vi "DivergeAngleScan.vi"(6 "Backgrund":T1, 7 "Session In":T2, 8 "俯仰CCD0":dbl, 10 "激光出口至CCD距离":dbl, 11 "旋转CCD0":dbl) -> (2 "近场图像":T1(plugin-control))   [LabVIEW 2018]
uses:
  <vilib>/userdefined/High Color/IMAQdx.ctl
  <vilib>/vision/Image Controls.llb/IMAQ Image.ctl
  <vilib>/vision/NI_Vision_Development_Module.lvlib
  <vilib>/vision/driver/NI_Vision_Acquisition_Software.lvlib
panel:
  out "近场相机.近场X范围":dbl
  out "近场相机.近场Y范围":dbl
  in  "停止":bool
  out "进度":dbl format="%05.2f%"
  out "YResolution":i32
  out "X Resolution":i32
  out "采集时间":u32
  out "运动时间":u32
  out "总时间":u32
  out "单步时间":u32
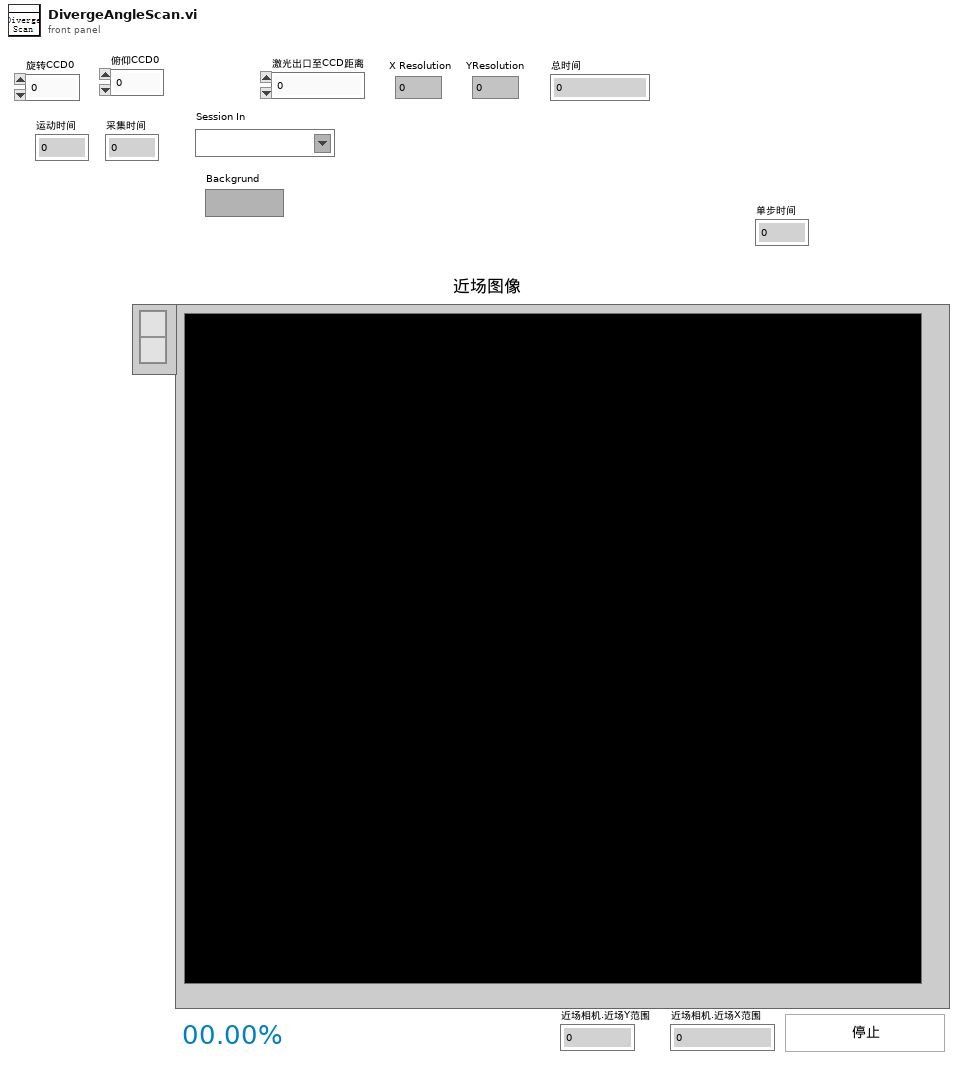
[diagram p1: front panel]
types:
  T1 = typedef "IMAQ Image.ctl" = refnum<image>
  T2 = typedef "IMAQdx.ctl" = refnum<k21>
  T3 = enum16{"计算总分辨率", "计算偏移量", "计算发散角分辨率", "计算发散角偏移量"}
  T4 = typedef "Image Type" = u32
  T5 = cluster{"示波器":cluster{"Channel (0:Channel 1)":enum16{"Channel 1", "Channel 2", "Channel 3", "Channel 4"}, "电压范围":dbl, "触发电压":dbl, "时间范围":dbl, " 示波器VISA":refnum<visa-resource-name>, "时间范围 标签":u64, "电压范围 标签":u64, "触发电压 标签":u64, "输入阻抗/Ω":u64}, "光谱仪":cluster{"SpecDataReference":refnum<queue>, "grating center":dbl, "Exposure Time (s)":dbl, "是否进行详细设置":bool, " 开始通信检查":bool, "通信成功？":bool, "波长":dbl}, " 近场相机":cluster{"曝光时间/us":dbl, "模拟增益":i32, "控制套接字":i32, "IP 地址":string, " 采集套接字":i32, "  版本号":i32, "ImageData":T1, "  增益最大":i32, "  增益最小":i32, " 曝光最大":i32, " 曝光最小":i32, " 帧速":i32, " 同步切换":i32, "  曝光缩放":i32, "Camera Source":refnum<k21>, "近场X范围":dbl, "近场Y范围":dbl, "单个像元大小/um":dbl, "相机距离原点位置":dbl[], "是否测量发散角":bool, "光束类型":bool}, " 偏振仪":cluster{"电压范围":u64, "触发电压":u64, "时间范围":u64, "波长范围":enum16{"可见光 400-700nm", "近红外 700-1100nm"}, "可见光偏振测量仪VISA":refnum<visa-resource-name>, "近红外偏振测量仪VISA":refnum<visa-resource-name>}, " 功率计":cluster{"通道":enum16{"Channel 1", "Channel 2"}, "工作波长":u32, "单位":u64, "时间范围":u64, "IP地址":string, "端口":u32, "是否需要散射片":bool}, "能量计":cluster{"通道":enum16{"Channel 1", "Channel 2"}, "工作波长":u32, "单位":u64, "时间范围":u64, "IP地址":string, "端口":u32, "能量计量程":enum16{"200uJ", "20uJ", "2uJ", "200nJ"}}, "电机":cluster{"Channel (0:Channel 1)":enum16{"Channel 1", "Channel 2", "Channel 3", "Channel 4"}, "电压范围":u64, "触发电压":u64, "时间范围":u64}, " 远场相机":cluster{"曝光时间":i32, "模拟增益":i32, "控制套接字":i32, "IP 地址":string, " 采集套接字":i32, "  版本号":i32, "ImageData":T1, "  增益最大":i32, "  增益最小":i32, " 曝光最大":i32, " 曝光最小":i32, " 帧速":i32, " 同步切换":i32, "  曝光缩放":i32, "ImageData B":T1}}
  T6 = typedef "控制电机枚举器.ctl" = enum16{"Z", "Y", "X", "发散角", "俯仰", "旋转"}
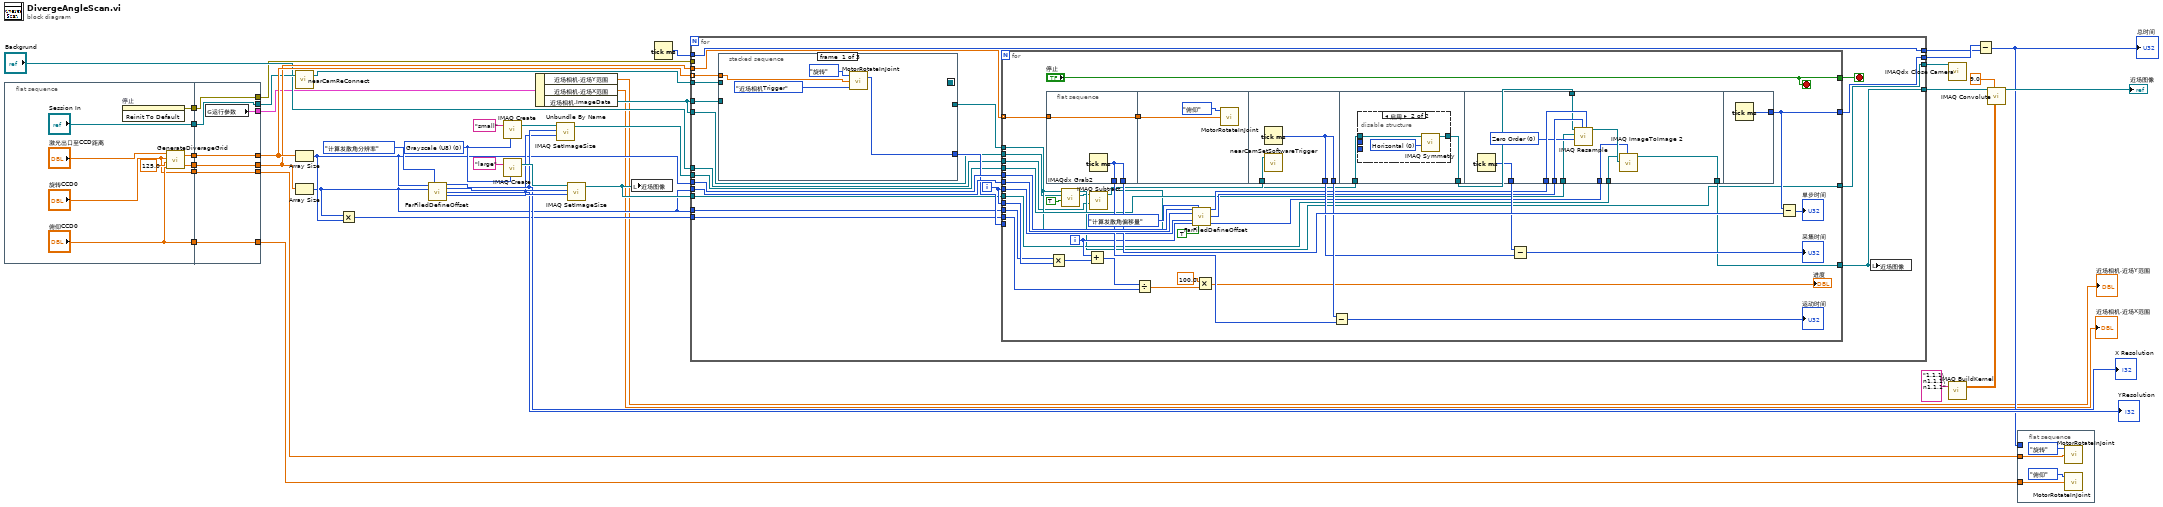
[diagram p0: block diagram]
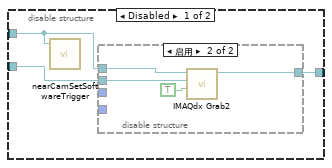
[diagram p4: hidden frame]
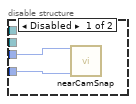
[diagram p5: hidden frame]
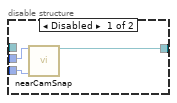
[diagram p6: hidden frame]
diagram:
  w28 = T4 0 items=["Grayscale (U8)", "Grayscale (I16)", "Grayscale (SGL)", "Complex (CSG)", "RGB (U32)", "HSL (U32)", "RGB (U64)", "Grayscale (U16)"] ("Image Type")
  n1 = flat-sequence {
    tunnel: [w49] -> w7
    tunnel: [w48] -> w6
    tunnel: ["俯仰CCD0"] -> w5
    tunnel: ["旋转CCD0"] -> w4
    tunnel: ["Session In"] -> w3
    tunnel: [w44] -> w2
    tunnel: [w53] -> w8
    tunnel: [w54] -> w13
    tunnel: [w55] -> w17
    tunnel: [w56] -> w18
    tunnel: [w57] -> w42
    tunnel: [w58] -> w43
    tunnel: w7 -> [w58]
    tunnel: w6 -> [w57]
    tunnel: w5 -> [w56]
    tunnel: w4 -> [w55]
    tunnel: w3 -> [w54]
    tunnel: w2 -> [w53]
    tunnel: [w52] -> w1
    frame #0 {
      n2 = invoke on="停止" class="Bool" method="Reinit To Default"() -> (error out=w44:errorcluster)  [unwired: 3 in, 2 out]
      n3 = call "GenerateDiverageGrid.vi"("俯仰CCD0"="俯仰CCD0", "TargetTheta"=125.0, "旋转CCD0"="旋转CCD0", "L"="激光出口至CCD距离") -> ("PitchGrid"=w48:dbl[], "RollGrid"=w49:dbl[])
    }
    frame #1 {
      n4 = global read "参数.vi" "运行参数"() -> (w52:T5)
    }
  }
  n5 = call "nearCamReConnect.vi"("Session In"=w13) -> ("IMAQdx Session Out"=w12:T2)  [unwired: 1 in, 1 out]
  n6 = Array Size(array=w43) -> (size(s)=w16:i32)
  n7 = Array Size(array=w42) -> (size(s)=w14:i32)
  n8 = Multiply(x=w14, y=w16) -> (x*y=w15:i32)
  n9 = call "FarFiledDefineOffset.vi"("X Pos Num"=w16, "状态"=T3."计算发散角分辨率", "Y Pos Num"=w14) -> ("单个分辨率X"=w21:i32, "X Resolution"=w39:i32, "单个分辨率Y"=w20:i32, "Y Resolution"=w38:i32)  [unwired: 8 in, 1 out]
  "X Resolution" <- w21
  "YResolution" <- w20
  n10 = call "IMAQ Create"("Image Name"="small", "Image Type"=w28) -> ("New Image"=w36:T1)  [unwired: 3 in, 1 out]
  n11 = call "IMAQ Create"("Image Name"="large", "Image Type"=w28) -> ("New Image"=w41:T1)  [unwired: 3 in, 1 out]
  n12 = Unbundle By Name(w1) -> ("近场相机.近场Y范围"=→"近场相机.近场Y范围":dbl, "近场相机.近场X范围"=→"近场相机.近场X范围":dbl, "近场相机.ImageData"=w22:T1)
  n13 = call "IMAQ SetImageSize"("Y Resolution"=w20, "X Resolution"=w21, "Image"=w36) -> ("Image Out"=w27:T1)  [unwired: 2 in, 1 out]
  n14 = call "IMAQ SetImageSize"("Y Resolution"=w38, "X Resolution"=w39, "Image"=w41) -> ("Image Out"=w24:T1)  [unwired: 2 in, 1 out]
  n15 = local write "近场图像"(w24) -> ()
  n16 = Tick Count (ms)() -> (millisecond timer value=w35:u32)
  n17 = for {
    tunnel: w43 -> [w68] mode=indexing
    tunnel: w42 -> [w67]
    tunnel: w27 -> [w61]
    tunnel: w24 -> [w60]
    tunnel: w16 -> [w78]
    tunnel: w14 -> [w77]
    tunnel: w35 -> [w75]
    tunnel: [w76] -> w34
    tunnel: [w75] -> w33
    tunnel: [w74] -> w29
    tunnel: w22 -> [w72]
    tunnel: [w71] -> w23
    tunnel: w12 -> [w70]
    tunnel: w22 -> [w69]
    tunnel: w15 -> [w65]
    tunnel: w14 -> [w63]
    tunnel: w8 -> [_]
    tunnel: "Backgrund" -> [w59]
    i -> [w64]
    stop <- w66 stop-if-true
    n18 = stacked-sequence {
      seq-local: [_ w83 _] -> [_ _ w84]
      tunnel: w68 -> [w81 _ _]
      tunnel: [w79 _ _] -> w73
      tunnel: w70 -> [_ w83 _]
      tunnel: w69 -> [_ _ w86]
      tunnel: [_ _ w85] -> w62
      frame #0 {
        n19 = call "MotorRotateInJoint.vi"("动作IO"=enum16{"近场相机Trigger", "远场相机Trigger"}."近场相机Trigger", "位置"=w81, "axis"=控制电机枚举器."旋转" ("控制电机")) -> ("返回"=w79:i32)  [unwired: 1 in]
      }
      frame #1 {
      }
      frame #2 {
        n20 = disable-structure shown="启用" {
          disable-tunnel: w86 -> [w89 _]
          disable-tunnel: [w88 w97] -> w85
          disable-tunnel: w84 -> [w87 w97]
          frame Disabled {
            n21 = call "nearCamSetSoftwareTrigger.vi"("IMAQdx Session"=w87) -> ()  [unwired: 3 in, 2 out]
            n22 = disable-structure shown="启用" {
              disable-tunnel: _ -> [w92 _]
              disable-tunnel: _ -> [w91 _]
              disable-tunnel: w89 -> [_ w96]
              disable-tunnel: w87 -> [_ w94]
              disable-tunnel: [_ w93] -> w88
              frame Disabled {
                n23 = call "nearCamSnap.vi"("采集套接字"=w92, "版本号"=w91) -> ("ImageData"=w90:T1)  [unwired: 9 in, 4 out]
              }
              frame Enabled {
                n24 = call <vilib>:"IMAQdx Grab2.vi"("Wait for Next Buffer? (Yes)"=TRUE, "Image In"=w96, "Session In"=w94) -> ("Session Out"=w93:T2)  [unwired: 5 in, 3 out]
              }
            }
          }
          frame Enabled {
          }
        }
      }
    }
    n25 = for {
      tunnel: w78 -> [w137]
      tunnel: w77 -> [w136]
      tunnel: w64 -> [w122]
      tunnel: [w105] -> w74
      tunnel: [w133] -> w76
      tunnel: w73 -> [_]
      tunnel: w72 -> [w101]
      tunnel: [w102] -> w71
      tunnel: w67 -> [w123] mode=indexing
      tunnel: ["停止"] -> w66
      tunnel: w65 -> [w120]
      tunnel: w64 -> [w119]
      tunnel: w63 -> [w118]
      tunnel: w62 -> [w103]
      tunnel: w61 -> [w109]
      tunnel: w60 -> [w106]
      tunnel: w59 -> [w98]
      i -> [w116]
      stop <- "停止" stop-if-true
      n26 = flat-sequence {
        tunnel: w123 -> [w139]
        tunnel: [w139] -> w135
        tunnel: [w138] -> w134
        tunnel: [w138] -> w128
        tunnel: w135 -> [w140]
        tunnel: [w143] -> w129
        tunnel: [w143] -> w125
        tunnel: w103 -> [w142]
        tunnel: [w145] -> w108
        tunnel: w99 -> [w144]
        tunnel: [w161] -> w126
        tunnel: w111 -> [w159]
        tunnel: w110 -> [w158]
        tunnel: w109 -> [w156]
        tunnel: w108 -> [w155]
        tunnel: w107 -> [w154]
        tunnel: w106 -> [w153]
        tunnel: [w152] -> w105
        tunnel: [w162] -> w133
        frame #0 {
          n27 = Tick Count (ms)() -> (millisecond timer value=w138:u32)
        }
        frame #1 {
          n28 = call "MotorRotateInJoint.vi"("位置"=w140, "axis"=控制电机枚举器."俯仰" ("控制电机")) -> ()  [unwired: 2 in, 1 out]
        }
        frame #2 {
          n29 = Tick Count (ms)() -> (millisecond timer value=w143:u32)
          n30 = call "nearCamSetSoftwareTrigger.vi"("IMAQdx Session"=w142) -> ()  [unwired: 3 in, 2 out]
        }
        frame #3 {
          n31 = disable-structure shown="启用" {
            disable-tunnel: [w148 w150] -> w145
            disable-tunnel: _ -> [w147 _]
            disable-tunnel: _ -> [w146 _]
            disable-tunnel: w144 -> [_ w149]
            frame Disabled {
              n32 = call "nearCamSnap.vi"("采集套接字"=w147, "版本号"=w146) -> ("Image Out"=w148:T1)  [unwired: 10 in, 3 out]
            }
            frame Enabled {
              w151 = u32 0 items=["Horizontal", "Vertical", "Central", "1st Diagonal", "2nd Diagonal"] ("Type of Symmetry")
              n33 = call "IMAQ Symmetry"("Type of Symmetry"=w151, "Image Src"=w149) -> ("Image Dst Out"=w150:T1)  [unwired: 3 in, 1 out]
            }
          }
        }
        frame #4 {
          w157 = u32 0 items=["Zero Order", "Bi-Linear", "Quadratic", "Cubic Spline"] ("Interpolation Type")
          n34 = Tick Count (ms)() -> (millisecond timer value=w161:u32)
          n35 = call "IMAQ Resample"("X Resolution"=w159, "Y Resolution"=w158, "Interpolation Type"=w157, "Image Dst"=w156, "Image Src"=w155) -> ("Image Dst Out"=w160:T1)  [unwired: 5 in, 1 out]
          n36 = call "IMAQ ImageToImage 2"("Offset Left/Top"=w154, "Image Src (Small)"=w160, "Image Src (Large)"=w153) -> ("Image Dst Out"=w152:T1)  [unwired: 7 in, 1 out]
        }
        frame #5 {
          n37 = Tick Count (ms)() -> (millisecond timer value=w162:u32)
        }
      }
      n38 = Multiply(x=w118, y=w119) -> (x*y=w117:i32)
      n39 = call <vilib>:"IMAQdx Grab2.vi"("Wait for Next Buffer? (Yes)"=TRUE, "Image In"=w101, "Session In"=w103) -> ("Image Out"=w100:T1, "Session Out"=w102:T2)  [unwired: 5 in, 2 out]
      n40 = Add(x=w116, y=w117) -> (x+y=w115:i32)
      n41 = call "IMAQ Subtract"("Image Src A"=w100, "Image Src B"=w98) -> ("Image Dst Out"=w99:T1)  [unwired: 5 in, 1 out]
      n42 = Divide(x=w115, y=w120) -> (x/y=w114:dbl)
      n43 = call "FarFiledDefineOffset.vi"("X Pos Num"=w137, "状态"=T3."计算发散角偏移量", "Y Pos Num"=w136, "当前X位置"=w122, "当前Y位置"=w116, "正序？"=TRUE) -> ("单个分辨率X"=w111:i32, "单个分辨率Y"=w110:i32, "offset"=w107:i32[])  [unwired: 5 in, 2 out]
      n44 = Multiply(x=100.0, y=w114) -> (x*y=→"进度":dbl)
      n45 = Subtract(x=w129, y=w128) -> (x-y=→"运动时间":u32)
      n46 = Subtract(x=w126, y=w125) -> (x-y=→"采集时间":u32)
      n47 = Subtract(x=w133, y=w134) -> (x-y=→"单步时间":u32)
    }
    n48 = local write "近场图像"(w74) -> ()
  }
  n49 = call <vilib>:"IMAQdx Close Camera.vi"("Session In"=w23) -> ()  [unwired: 10 in, 1 out]
  n50 = call "IMAQ BuildKernel"("Kernel String"="1,1,1\n1,1,1\n1,1,1") -> ("Kernel"=w30:sgl[][])  [unwired: 4 in, 1 out]
  n51 = Subtract(x=w34, y=w33) -> (x-y=w19:u32)
  "总时间" <- w19
  n52 = call "IMAQ Convolute"("Kernel"=w30, "Divider (kernel sum)"=sgl 9.0, "Image Src"=w29) -> ("Image Dst Out"=→"近场图像":T1)  [unwired: 7 in, 1 out]
  n53 = flat-sequence {
    tunnel: w19 -> [_]
    tunnel: w18 -> [w164]
    tunnel: w17 -> [w163]
    frame #0 {
      n54 = call "MotorRotateInJoint.vi"("位置"=w163, "axis"=控制电机枚举器."旋转" ("控制电机")) -> ()  [unwired: 2 in, 1 out]
      n55 = call "MotorRotateInJoint.vi"("位置"=w164, "axis"=控制电机枚举器."俯仰" ("控制电机")) -> ()  [unwired: 2 in, 1 out]
    }
  }
